vi "Mätning av ytresistivitet.vi"() -> ()   [LabVIEW 2024]
panel:
  out "Ytresistivitet, mWm":dbl
  out "Ytresistans, mW/*":dbl
  out "Mätvärden":dbl[][](array[numeric])
  out "% - max/min":dbl
  out "Max, Ytresistivitet":dbl
  out "Max, Ytresistans":dbl
  out "Min, Ytresistans":dbl
  out "Min, Ytresistivitet":dbl
  in  "Rensa sparade värden":bool
  in  "?":enum32{"Visa", "Göm"}(tab)
  out "Mätvärden2":dbl[][](array[numeric])
  out "% - skillnad":dbl
  out "Min":dbl format="%#_13g"
  out "Max":dbl
  out "Spänning.cal":dbl
  out "Ström.cal":dbl
  out "Redo för mätning3":bool
  out "Redo för mätning2":bool
  out "Redo för mätning":bool
  out "Mätning pågår":bool
  out "Kalibrering pågår":bool
  in  "Tab Control":T1(tab)
  in  "cal_onoff":bool caption="Boolean"
  in  "Sätt ström":bool
  in  "Nollställ ström":bool
  in  "Ange strömmen, mA":dbl
  in  "Kva/Lin":bool caption="Boolean"
  in  "Tjocklek, um":dbl
  in  "Material":string
  in  "Spänningsaggregat":refnum<visa-resource-name>="COM1"
  in  "Spänningsmultimeter":refnum<visa-resource-name>="USB0::0x0957::0x1B07::MY53100226::INSTR"
  in  "Strömmultimeter":refnum<visa-resource-name>="USB0::0x0957::0x1A07::MY53201212::INSTR"
  in  "Spara mätdata i textfil - linjärt":path
  in  "Spara mätdata i textfil - kvadratiskt":path
  in  "Spänning (V) +/- för kalibrering, default = 0,01V":dbl
  in  "Mapp för excelfiler":path=path "\\\\filur03.it.liu.se\\students/axefr422/Documents/Labview program/excel"
  in  "Samples/mätning, default = 10":i32
  in  "Max spänning (V), default = 1":dbl
  in  "Starta mätning":bool=TRUE
  in  "stop":bool
  # "Mätvärden"
  # "Medelvärden"
  # "Ytresistans, mW/*"
  # "Ytresistivitet, mWm"
  # "Specifik mätdata - Aktuell mätning"
  # "Spänning, V"
  # "Ström, A"
  # "Ytresistivitet, mWm"
  # "Ytresistans, mW/sq"
  # "Ytresistans"
  # "Kvadratiskt"
  # "Linjärt"
  # "Kalibrering av"
  # "Kalibrering på"
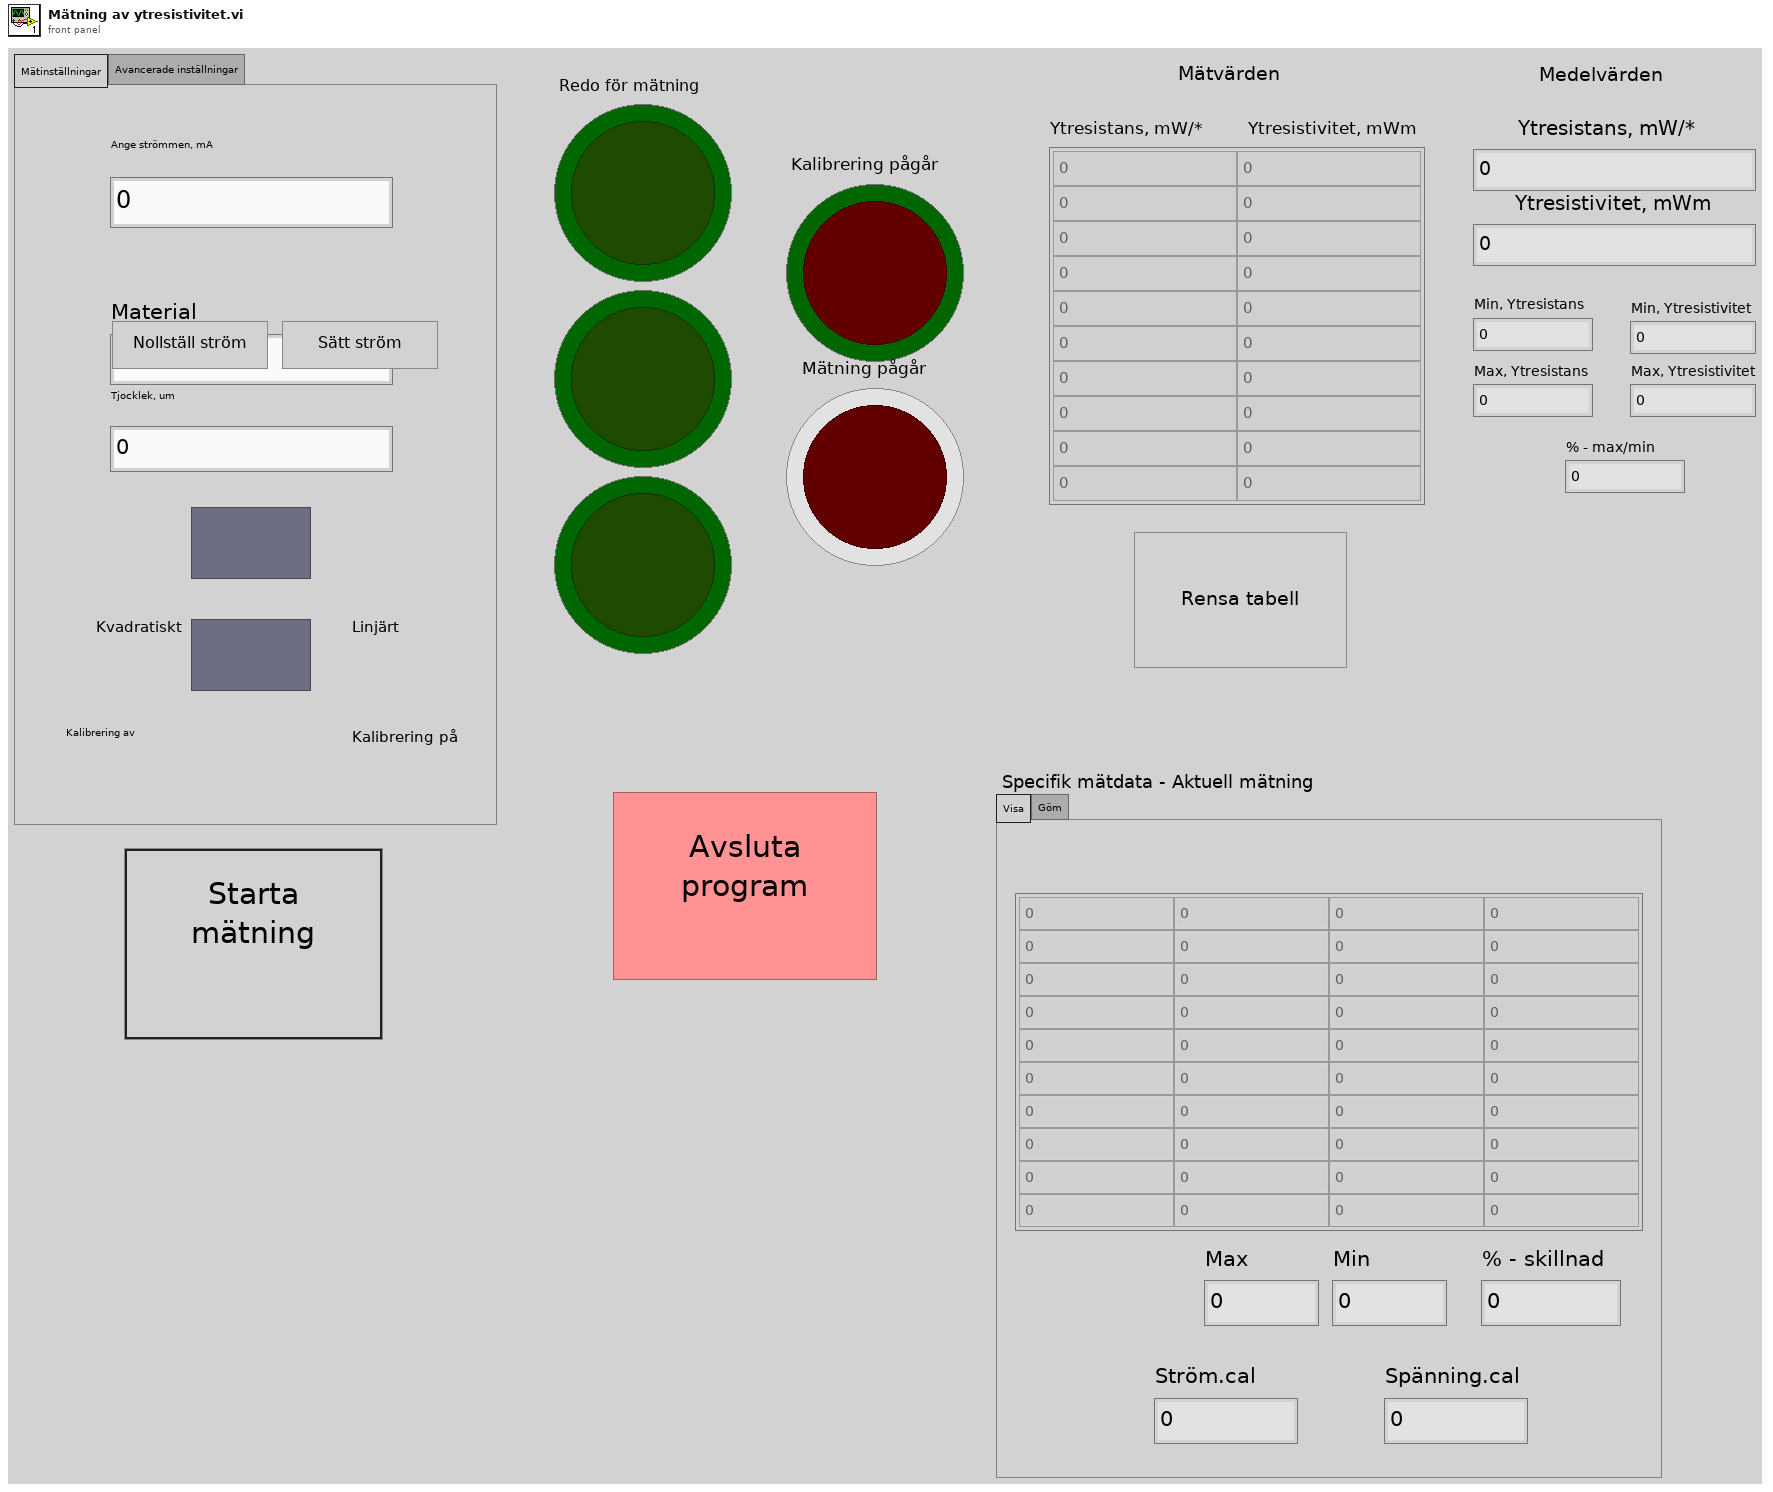
[diagram p1: front panel]
types:
  T1 = enum32{"Mätinställningar", "Avancerade inställningar"}
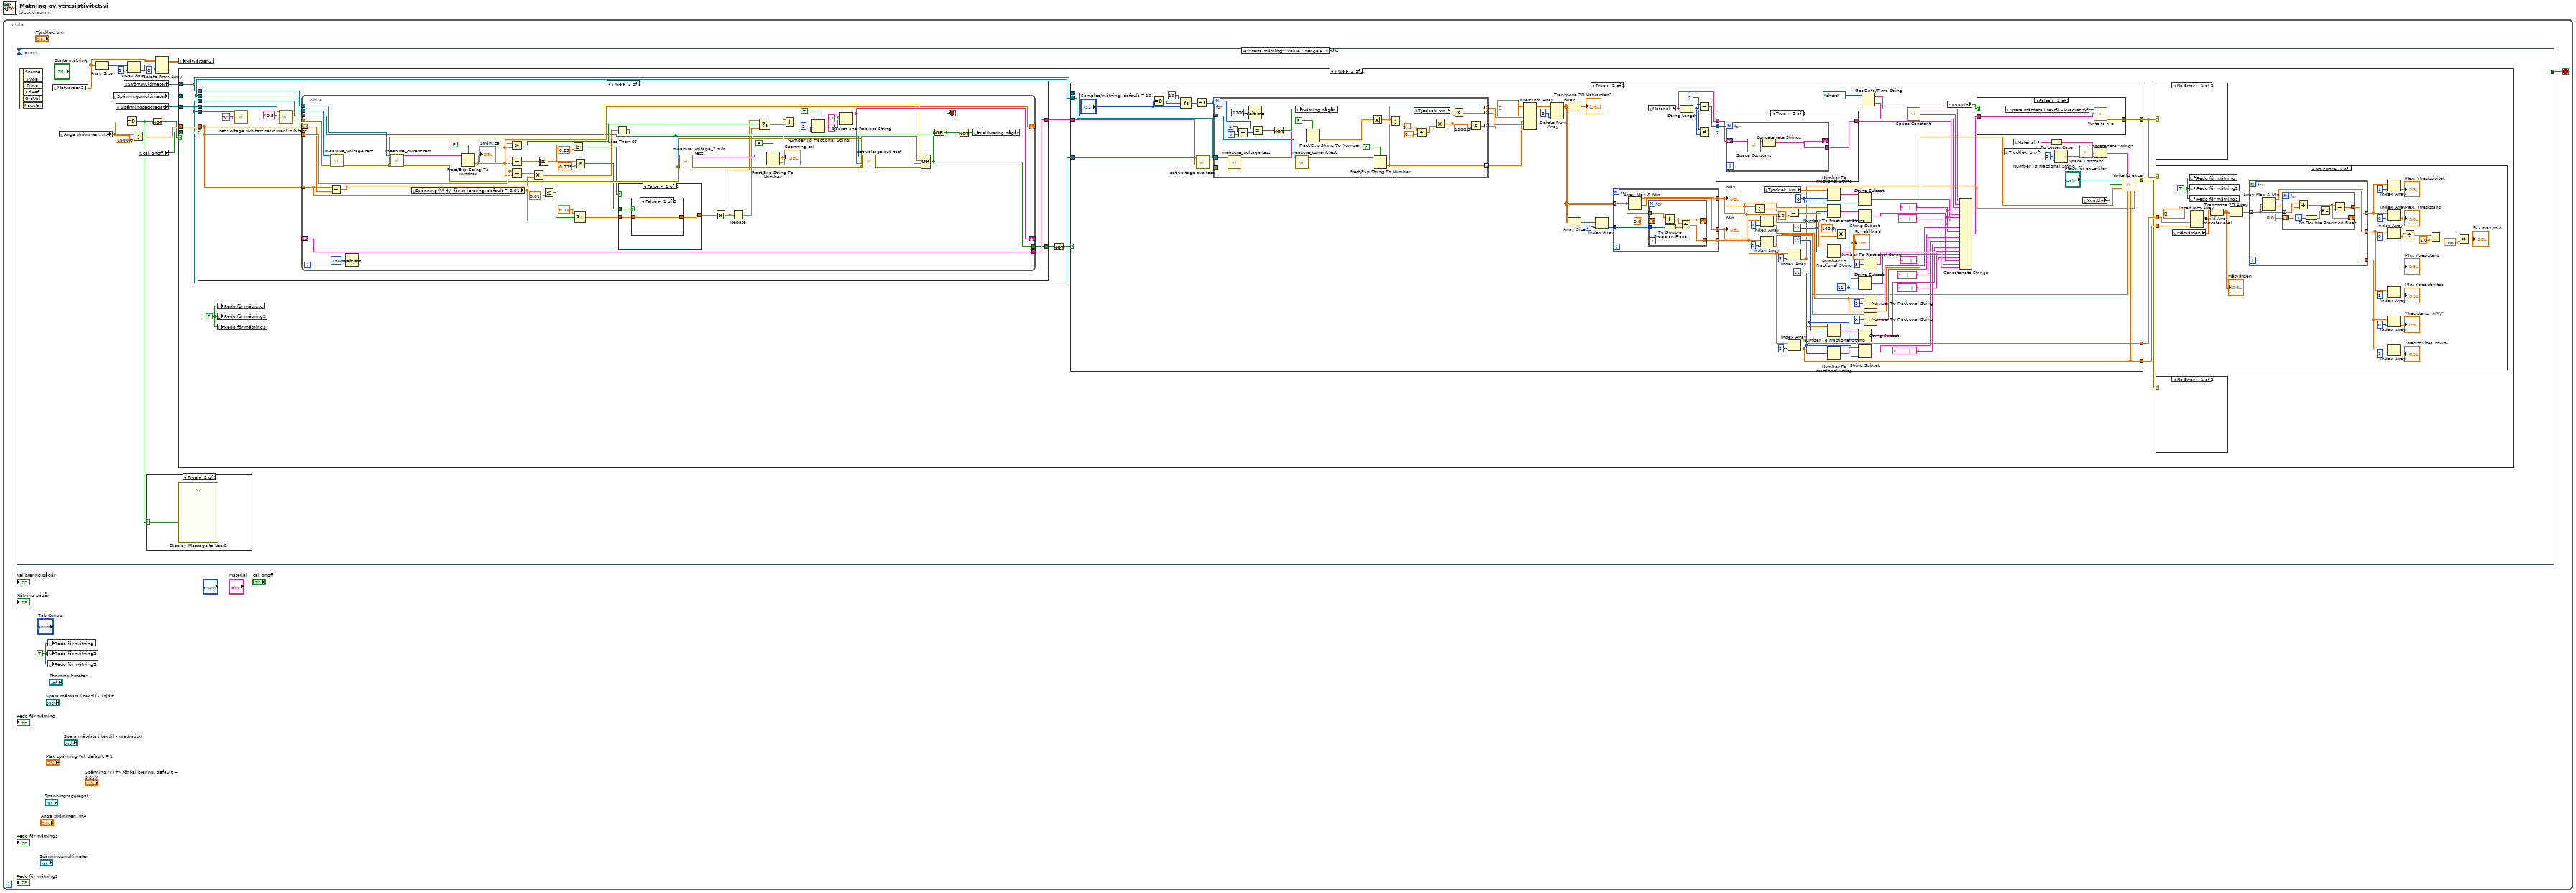
[diagram p0: block diagram]
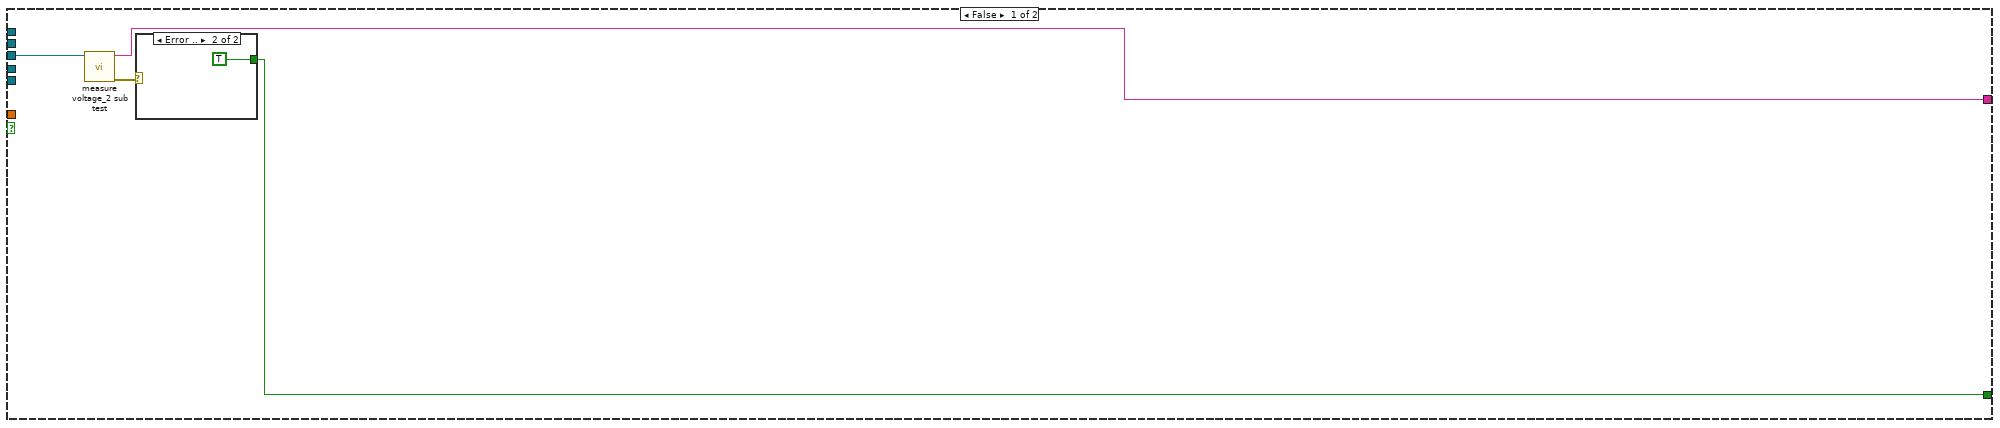
[diagram p4: hidden frame]
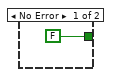
[diagram p5: hidden frame]
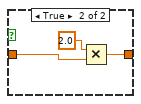
[diagram p6: hidden frame]
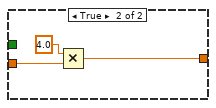
[diagram p7: hidden frame]
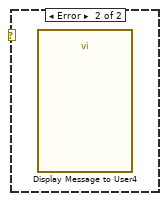
[diagram p8: hidden frame]
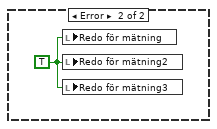
[diagram p9: hidden frame]
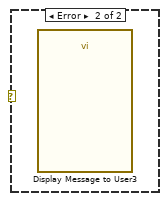
[diagram p10: hidden frame]
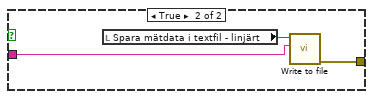
[diagram p12: hidden frame]
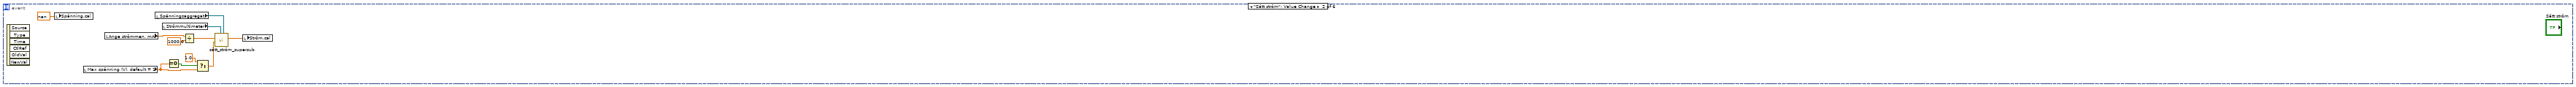
[diagram p14: hidden frame]
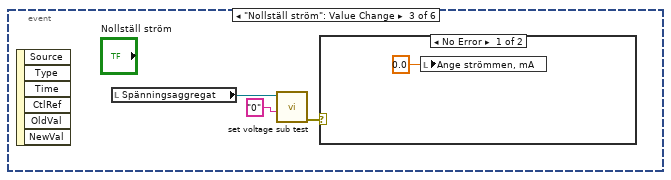
[diagram p15: hidden frame]
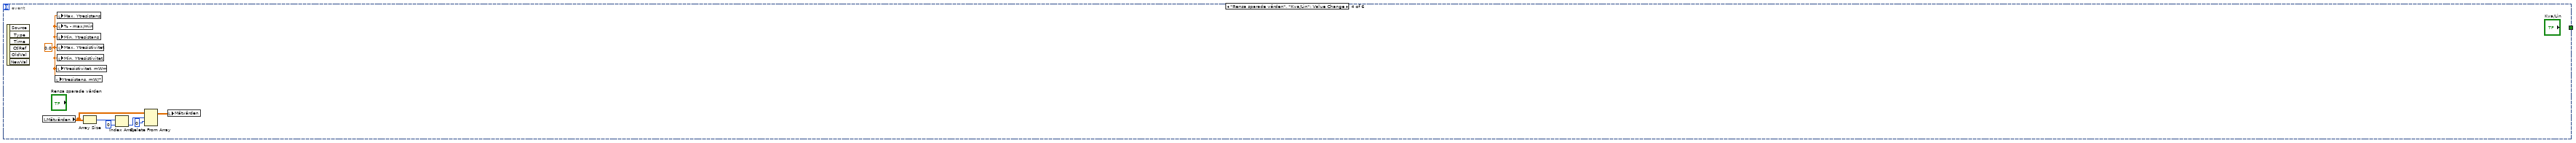
[diagram p17: hidden frame]
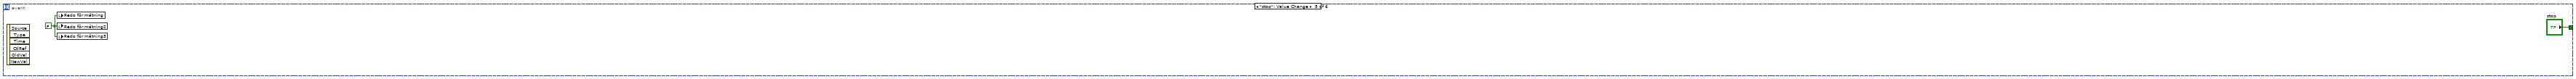
[diagram p18: hidden frame]
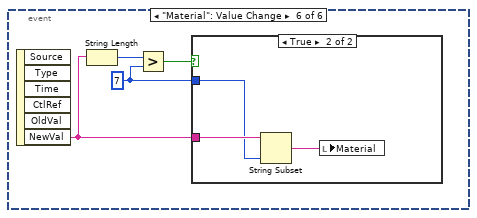
[diagram p19: hidden frame]
diagram:
  n1 = while {
    stop <- w2 stop-if-true
    w1 = TRUE ("Redo för mätning")
    n2 = event shown="[0] \"Starta mätning\": Value Change" {
      selector: _ -> [_ _ _ _ _ _]
      dyn-events: _ -> [_ _ _ _ _ _]
      timeout: _ -> [_ _ _ _ _ _]
      tunnel: [_ _ _ _ "stop" _] -> w2
      event "Starta mätning": Value Change {
        n3 = event-data() -> ()  [unwired: 1 in, 6 out]
        n4 = local read "Mätvärden2"() -> (w6:dbl[][])
        n5 = local read "Ange strömmen, mA"() -> (w12:dbl)
        n6 = Array Size(array=w6) -> (size(s)=w9:i32[])
        n7 = local read "Spänningsmultimeter"() -> (w14:refnum<visa-resource-name>)
        n8 = local read "Spänningsaggregat"() -> (w15:refnum<visa-resource-name>)
        n9 = local read "Strömmultimeter"() -> (w13:refnum<visa-resource-name>)
        n10 = Equal To 0?(x=w12) -> (x = 0?=w11:bool)
        n11 = Index Array(array=w9, index=0) -> (element=w7:i32)
        n12 = Divide(x=w12, y=1000.0) -> (x/y=w16:dbl)
        n13 = local read "cal_onoff"() -> (w3:bool)
        n14 = case shown="True" w11 {
          selector: w11 -> [_ w18]
          frame False {
          }
          frame True {
            n15 = call "Display Message to User2"("Enable"=w18) -> ()  [unwired: 9 in, 2 out]
          }
        }
        n16 = Not(x=w11) -> (.not. x?=w10:bool)
        n17 = Delete From Array(array=w6, length=w7, index (row)=0) -> (array with subset deleted=w5:dbl[][])  [unwired: 1 in, 1 out]
        n18 = local write "Mätvärden2"(w5) -> ()
        n19 = case shown="True" w10 {
          tunnel: w16 -> [_ w26]
          tunnel: w15 -> [_ w20]
          tunnel: w14 -> [_ w31]
          tunnel: w13 -> [_ w30]
          tunnel: w3 -> [_ w21]
          frame False {
          }
          frame True {
            w19 = FALSE ("Redo för mätning")
            n20 = case shown="True" w21 {
              tunnel: w31 -> [_ w49]
              tunnel: w30 -> [_ w48]
              tunnel: [w34 w47] -> w29
              tunnel: w20 -> [w35 w46]
              tunnel: [w32 w45] -> w28
              tunnel: w26 -> [_ w44]
              tunnel: w20 -> [_ w42]
              tunnel: w20 -> [_ w40]
              frame False {
                n21 = call "measure voltage_2 sub test.vi"("VISA Refnum in"=w35) -> ("error out"=w33:errorcluster, "Reponse"=w34:string)  [unwired: 9 in]
                n22 = case shown="Error .." w33 {
                  tunnel: [FALSE TRUE] -> w32
                  frame No Error {
                  }
                  frame Error {
                  }
                }
              }
              frame True {
                n23 = call "set voltage sub test.vi"("result string"="0", "VISA Refnum in"=w42) -> ("error out"=w43:errorcluster)  [unwired: 9 in]
                n24 = call "set current sub test.vi"("error in (no error)"=w43, "result string"="0.5", "VISA Refnum in"=w40) -> ("error out"=w39:errorcluster)  [unwired: 8 in]
                n25 = while {
                  tunnel: w44 -> [w98]
                  shift-right: [w67] -> _
                  shift-left: w44 -> [w96]
                  shift-right: [w97] -> _
                  shift-left: _ -> [w95]
                  tunnel: [w95] -> w47
                  tunnel: w46 -> [w51]
                  tunnel: w49 -> [w52]
                  tunnel: w48 -> [w76]
                  tunnel: [w70] -> w45
                  tunnel: w44 -> [w68]
                  tunnel: w39 -> [w50]
                  stop <- w71 stop-if-true
                  n26 = Subtract(x=w68, y=w96) -> (x-y=w85:dbl)
                  n27 = call "measure_voltage test.vi"("error in (no error)"=w50, "VISA Refnum in"=w52) -> ("error out"=w75:errorcluster)  [unwired: 8 in, 1 out]
                  n28 = Wait (ms)(milliseconds to wait=u32 750) -> ()  [unwired: 1 out]
                  n29 = call "measure_current test.vi"("error in (no error)"=w75, "VISA Refnum in"=w76) -> ("error out"=w74:errorcluster, "read buffer"=w78:string)  [unwired: 8 in]
                  n30 = local read "Spänning (V) +/- för kalibrering, default = 0,01V"() -> (w54:dbl)
                  n31 = Fract/Exp String To Number(use system decimal point (T)=FALSE, string=w78) -> (number=w67:dbl)  [unwired: 2 in, 1 out]
                  "Ström.cal" <- w67
                  n32 = Greater Or Equal?(x=w98, y=w67) -> (x >= y?=w92:bool)
                  n33 = Subtract(x=w68, y=w67) -> (x-y=w66:dbl)
                  n34 = Subtract(x=w68, y=w67) -> (x-y=w84:dbl)
                  n35 = Multiply(x=w84, y=w85) -> (x*y=w86:dbl)
                  n36 = Absolute Value(x=w66) -> (abs(x)=w58:dbl)
                  n37 = Less Or Equal?(x=w54, y=0.01) -> (x <= y?=w55:bool)
                  n38 = Greater Or Equal?(x=w58, y=0.25) -> (x >= y?=w64:bool)
                  n39 = Select(t=0.01, s=w55, f=w54) -> (s? t:f=w56:dbl)
                  n40 = Greater Or Equal?(x=w58, y=0.075) -> (x >= y?=w60:bool)
                  n41 = Less Than 0?(x=w86) -> (x < 0?=w72:bool)
                  n42 = case shown="False" w64 {
                    tunnel: w56 -> [w100 w108]
                    tunnel: [w99 w106] -> w63
                    tunnel: w60 -> [w101 _]
                    frame False {
                      n43 = case shown="False" w101 {
                        tunnel: w100 -> [w102 w104]
                        tunnel: [w102 w103] -> w99
                        frame False {
                        }
                        frame True {
                          n44 = Multiply(x=2.0, y=w104) -> (x*y=w103:dbl)
                        }
                      }
                    }
                    frame True {
                      n45 = Multiply(x=4.0, y=w108) -> (x*y=w106:dbl)
                    }
                  }
                  n46 = call "measure voltage_2 sub test.vi"("error in (no error)"=w74, "VISA Refnum in"=w51) -> ("error out"=w73:errorcluster, "Reponse"=w79:string)  [unwired: 8 in]
                  n47 = Absolute Value(x=w63) -> (abs(x)=w61:dbl)
                  n48 = Negate(x=w61) -> (-x=w62:dbl)
                  n49 = Select(t=w61, s=w92, f=w62) -> (s? t:f=w91:dbl)
                  n50 = Fract/Exp String To Number(use system decimal point (T)=FALSE, string=w79) -> (number=w81:dbl)  [unwired: 2 in, 1 out]
                  "Spänning.cal" <- w81
                  n51 = Add(x=w81, y=w91) -> (x+y=w83:dbl)
                  n52 = Number To Fractional String(use system decimal point (T)=TRUE, number=w83, precision (6)=i16 2) -> (F-format string=w82:string)  [unwired: 1 in]
                  n53 = Search and Replace String(input string=w82, search string=",", replace string="." ("replace string (\"\")")) -> (result string=w97:string)  [unwired: 5 in, 3 out]
                  n54 = call "set voltage sub test.vi"("error in (no error)"=w73, "result string"=w97, "VISA Refnum in"=w51) -> ("error out"=w69:errorcluster)  [unwired: 8 in]
                  n55 = Compound Arithmetic op=OR(w75, w74, w73, w69) -> (w70:bool)
                  n56 = Or(x=w70, y=w72) -> (x .or. y?=w71:bool)
                  n57 = Not(x=w71) -> (.not. x?=w77:bool)
                  n58 = local write "Kalibrering pågår"(w77) -> ()
                }
              }
            }
            n59 = local write "Redo för mätning"(w19) -> ()
            n60 = local write "Redo för mätning2"(w19) -> ()
            n61 = local write "Redo för mätning3"(w19) -> ()
            n62 = Not(x=w28) -> (.not. x?=w27:bool)
            n63 = case shown="True" w27 {
              tunnel: w31 -> [_ w179]
              tunnel: w30 -> [_ w178]
              tunnel: w29 -> [_ w177]
              tunnel: w20 -> [_ w176]
              tunnel: [_ w174] -> w25
              tunnel: [_ w162] -> w23
              tunnel: [_ w161] -> w24
              tunnel: [_ w158] -> w22
              frame False {
              }
              frame True {
                w175 = i16 8 ("width (-)")
                w203 = i16 11 ("width (-)")
                w200 = i16 11 ("width (-)")
                w201 = 7 ("x")
                w199 = 11 ("length (rest)")
                w196 = i16 11 ("width (-)")
                w190 = "    |    "
                n64 = Equal To 0?(x="Samples/mätning, default = 10") -> (x = 0?=w156:bool)
                n65 = Select(t=10, s=w156, f="Samples/mätning, default = 10") -> (s? t:f=w153:i32)
                n66 = Increment(x=w153) -> (x+1=w157:i32)
                n67 = call "set voltage sub test.vi"("result string"=w177, "VISA Refnum in"=w176) -> ("error out"=w206:errorcluster)  [unwired: 9 in]
                n68 = for {
                  N: w157 -> [w282]
                  tunnel: [w269] -> w204 mode=indexing
                  tunnel: [w287] -> w205 mode=indexing
                  tunnel: w206 -> [w284]
                  tunnel: w179 -> [w276]
                  tunnel: w178 -> [w275]
                  tunnel: [w271] -> w221 mode=indexing
                  tunnel: [w264] -> w232 mode=indexing
                  i -> [w281]
                  n69 = call "measure_voltage test.vi"("error in (no error)"=w284, "VISA Refnum in"=w276) -> ("error out"=w283:errorcluster, "read buffer"=w285:string)  [unwired: 8 in]
                  n70 = Add(x=1, y=w281) -> (x+y=w277:i32)
                  n71 = Wait (ms)(milliseconds to wait=u32 1000) -> ()  [unwired: 1 out]
                  n72 = Equal?(x=w282, y=w277) -> (x = y?=w279:bool)
                  n73 = Not(x=w279) -> (.not. x?=w278:bool)
                  n74 = local write "Mätning pågår"(w278) -> ()
                  n75 = call "measure_current test.vi"("error in (no error)"=w283, "VISA Refnum in"=w275) -> ("read buffer"=w286:string)  [unwired: 8 in, 1 out]
                  n76 = Fract/Exp String To Number(use system decimal point (T)=FALSE, string=w285) -> (number=w270:dbl)  [unwired: 2 in, 1 out]
                  n77 = Absolute Value(x=w270) -> (abs(x)=w269:dbl)
                  n78 = Fract/Exp String To Number(use system decimal point (T)=FALSE, string=w286) -> (number=w287:dbl)  [unwired: 2 in, 1 out]
                  n79 = Divide(x=w269, y=w287) -> (x/y=w268:dbl)
                  n80 = local read "Tjocklek, um"() -> (w267:dbl)
                  n81 = Divide(x=3.141592653589793, y=0.6931471805599453) -> (x/y=w274:dbl)
                  n82 = Multiply(x=w268, y=w274) -> (x*y=w265:dbl)
                  n83 = Multiply(x=w267, y=w265) -> (x*y=w271:dbl)
                  n84 = Multiply(x=w265, y=1000.0) -> (x*y=w264:dbl)
                }
                n85 = Insert Into Array(array=dbl[][] [], new element #1=w204, new element #2=w205, new element #3=w221, new element #4=w232) -> (w207:dbl[][])  [unwired: 2 in]
                n86 = Delete From Array(array=w207, index (col)=0) -> (array with subset deleted=w215:dbl[][])  [unwired: 2 in, 1 out]
                n87 = Transpose 2D Array(2D array=w215) -> (transposed array=→"Mätvärden2":dbl[][])
                n88 = Array Size(array=w215) -> (size(s)=w208:i32[])
                n89 = Index Array(array=w208, index=1) -> (element=w209:i32)
                n90 = for {
                  tunnel: [w257] -> w234 mode=indexing
                  tunnel: w215 -> [w254] mode=indexing
                  tunnel: w209 -> [w255]
                  tunnel: [w253] -> w152
                  tunnel: [w252] -> w151
                  n91 = Array Max & Min(array=w254) -> (max value=w253:dbl, min value=w252:dbl)  [unwired: 2 out]
                  n92 = for {
                    tunnel: [w258] -> w257
                    shift-right: [w263] -> _
                    shift-left: 0.0 -> [w262]
                    tunnel: w254 -> [w260] mode=indexing
                    tunnel: w255 -> [w259]
                    n93 = Add(x=w260, y=w262) -> (x+y=w263:dbl)
                    n94 = To Double Precision Float(number=w259) -> (double precision float=w261:dbl)
                    n95 = Divide(x=w263, y=w261) -> (x/y=w258:dbl)
                  }
                }
                "Max" <- w152
                "Min" <- w151
                n96 = local read "Material"() -> (w227:string)
                n97 = String Length(string=w227) -> (length=w231:i32)
                n98 = Subtract(x=w201, y=w231) -> (x-y=w230:i32)
                n99 = Not Equal?(x=w201, y=w231) -> (x != y?=w229:bool)
                n100 = case shown="True" w229 {
                  tunnel: w230 -> [_ w248]
                  tunnel: w227 -> [w245 w247]
                  tunnel: [w245 w246] -> w228
                  frame False {
                  }
                  frame True {
                    n101 = for {
                      N: w248 -> [_]
                      shift-right: [w249] -> _
                      shift-left: w247 -> [w250]
                      tunnel: [w249] -> w246
                      n102 = call <vilib>:"Space Constant.vi"() -> ("String"=w251:string)
                      n103 = Concatenate Strings(w250, w251) -> (w249:string)
                    }
                  }
                }
                n104 = Divide(x=w152, y=w151) -> (x/y=w210:dbl)
                n105 = Index Array(array=w234, index=0) -> (element=w171:dbl)
                n106 = Index Array(array=w234, index=1) -> (element=w170:dbl)
                n107 = local read "Tjocklek, um"() -> (w222:dbl)
                n108 = Subtract(x=w210, y=1.0) -> (x-y=w214:dbl)
                n109 = Index Array(array=w234, index=3) -> (element=w162:dbl)
                n110 = Index Array(array=w234, index=2) -> (element=w161:dbl)
                n111 = Number To Fractional String(number=w222, precision (6)=w175) -> (F-format string=w223:string)  [unwired: 2 in]
                n112 = Number To Fractional String(number=w152, width (-)=w196) -> (F-format string=w218:string)  [unwired: 2 in]
                n113 = Number To Fractional String(number=w151, width (-)=w196) -> (F-format string=w217:string)  [unwired: 2 in]
                n114 = Number To Fractional String(number=w162, width (-)=w203) -> (F-format string=w233:string)  [unwired: 2 in]
                n115 = Number To Fractional String(number=w161, width (-)=w200) -> (F-format string=w219:string)  [unwired: 2 in]
                n116 = Multiply(x=100.0, y=w214) -> (x*y=w150:dbl)
                "% - skillnad" <- w150
                n117 = String Subset(string=w223, length (rest)=w175) -> (substring=w173:string)  [unwired: 1 in]
                n118 = String Subset(string=w218, length (rest)=w199) -> (substring=w237:string)  [unwired: 1 in]
                n119 = String Subset(string=w217, length (rest)=w199) -> (substring=w236:string)  [unwired: 1 in]
                n120 = String Subset(string=w233, length (rest)=w203) -> (substring=w235:string)  [unwired: 1 in]
                n121 = String Subset(string=w219, length (rest)=w200) -> (substring=w220:string)  [unwired: 1 in]
                n122 = Get Date/Time String(date format (0)=enum16{"short", "long", "abbreviated"}."short") -> (date string=w224:string, time string=w226:string)  [unwired: 2 in]
                n123 = Number To Fractional String(number=w150, width (-)=i16 8) -> (F-format string=w238:string)  [unwired: 2 in]
                n124 = Number To Fractional String(number=w171, width (-)=i16 9) -> (F-format string=w212:string)  [unwired: 2 in]
                n125 = Number To Fractional String(number=w170, width (-)=i16 8) -> (F-format string=w213:string)  [unwired: 2 in]
                n126 = call <vilib>:"Space Constant.vi"() -> ("String"=w225:string)
                n127 = local read "Kva/Lin"() -> (w160:bool)
                n128 = Concatenate Strings(w224, w225, w226, w190, w228, w190, w173, w190, w212, w190, w213, "    |      ", w220, "         |     ", w235, "       |   " ("string"), w236, "     |   " ("string"), w237, "     |    " ("string"), w238) -> (w211:string)
                n129 = case shown="False" w160 {
                  tunnel: w211 -> [w241 w243]
                  tunnel: [w239 w242] -> w174
                  frame False {
                    n130 = local read "Spara mätdata i textfil - kvadratiskt"() -> (w240:path)
                    n131 = call "Write to file.vi"("input string"=w241, "file path"=w240) -> ("error out"=w239:errorcluster)  [unwired: 9 in]
                  }
                  frame True {
                    n132 = local read "Spara mätdata i textfil - linjärt"() -> (w244:path)
                    n133 = call "Write to file.vi"("input string"=w243, "file path"=w244) -> ("error out"=w242:errorcluster)  [unwired: 9 in]
                  }
                }
                n134 = local read "Tjocklek, um"() -> (w165:dbl)
                n135 = local read "Material"() -> (w168:string)
                n136 = To Lower Case(string=w168) -> (all lower case string=w169:string)
                n137 = Number To Fractional String(number=w165, precision (6)=i16 2) -> (F-format string=w163:string)  [unwired: 2 in]
                n138 = call <vilib>:"Space Constant.vi"() -> ("String"=w166:string)
                n139 = local read "Kva/Lin"() -> (w159:bool)
                n140 = Concatenate Strings(w169, w166, w163) -> (w172:string)
                n141 = call "Write to excel.vi"("Mapp"="Mapp för excelfiler", "Filnamn"=w172, "Boolean"=w159, "Spänning"=w171, "Ström"=w170, "Ytresistivitet"=w161, "Ytresistans"=w162) -> ("error out"=w158:errorcluster)  [unwired: 2 in]
              }
            }
            n142 = case shown="No Error" w25 {
              frame No Error {
              }
              frame Error {
                n143 = call "Display Message to User3"() -> ()  [unwired: 10 in, 2 out]
              }
            }
            n144 = case shown="No Error" w25 {
              tunnel: w24 -> [w130 _]
              tunnel: w23 -> [w131 _]
              frame No Error {
                w109 = TRUE ("Redo för mätning")
                n145 = local read "Mätvärden"() -> (w128:dbl[][])
                n146 = local write "Redo för mätning"(w109) -> ()
                n147 = local write "Redo för mätning2"(w109) -> ()
                n148 = local write "Redo för mätning3"(w109) -> ()
                n149 = Insert Into Array(array=dbl[] [], new element #1=w131, new element #2=w130) -> (w127:dbl[])  [unwired: 1 in]
                n150 = Build Array (concatenate)(w128, w127) -> (w126:dbl[][])
                "Mätvärden" <- w126
                n151 = Transpose 2D Array(2D array=w126) -> (transposed array=w125:dbl[][])
                n152 = for {
                  tunnel: [w140] -> w134 mode=indexing
                  tunnel: w125 -> [w139] mode=indexing
                  tunnel: [w138] -> w123 mode=indexing
                  tunnel: [w137] -> w124 mode=indexing
                  n153 = Array Max & Min(array=w139) -> (max value=w138:dbl, min value=w137:dbl)  [unwired: 2 out]
                  n154 = for {
                    shift-right: [w145] -> _
                    shift-left: 0.0 -> [w148]
                    tunnel: [w146] -> w140
                    tunnel: w139 -> [w144] mode=indexing
                    i -> [w147]
                    n155 = Add(x=w144, y=w148) -> (x+y=w145:dbl)
                    n156 = To Double Precision Float(number=w147) -> (double precision float=w143:dbl)
                    n157 = Increment(x=w143) -> (x+1=w142:dbl)
                    n158 = Divide(x=w145, y=w142) -> (x/y=w146:dbl)
                  }
                }
                n159 = Index Array(array=w123, index=1) -> (element=→"Max, Ytresistivitet":dbl)
                n160 = Index Array(array=w123, index=0) -> (element=w118:dbl)
                "Max, Ytresistans" <- w118
                n161 = Index Array(array=w124, index=0) -> (element=w117:dbl)
                "Min, Ytresistans" <- w117
                n162 = Index Array(array=w124, index=1) -> (element=→"Min, Ytresistivitet":dbl)
                n163 = Index Array(array=w134, index=0) -> (element=→"Ytresistans, mW/*":dbl)
                n164 = Index Array(array=w134, index=1) -> (element=→"Ytresistivitet, mWm":dbl)
                n165 = Divide(x=w118, y=w117) -> (x/y=w116:dbl)
                n166 = Subtract(x=w116, y=1.0) -> (x-y=w114:dbl)
                n167 = Multiply(x=w114, y=100.0) -> (x*y=→"% - max/min":dbl)
              }
              frame Error {
                w149 = TRUE ("Redo för mätning3")
                n168 = local write "Redo för mätning"(w149) -> ()
                n169 = local write "Redo för mätning2"(w149) -> ()
                n170 = local write "Redo för mätning3"(w149) -> ()
              }
            }
            n171 = case shown="No Error" w22 {
              frame No Error {
              }
              frame Error {
                n172 = call "Display Message to User4"() -> ()  [unwired: 10 in, 2 out]
              }
            }
          }
        }
      }
      event "Sätt ström": Value Change {
        n173 = event-data() -> ()  [unwired: 1 in, 6 out]
        n174 = local write "Spänning.cal"(nan ("Spänning.cal")) -> ()
        n175 = local read "Max spänning (V), default = 1"() -> (w295:dbl)
        n176 = local read "Ange strömmen, mA"() -> (w300:dbl)
        n177 = local read "Spänningsaggregat"() -> (w293:refnum<visa-resource-name>)
        n178 = local read "Strömmultimeter"() -> (w301:refnum<visa-resource-name>)
        n179 = Equal To 0?(x=w295) -> (x = 0?=w297:bool)
        n180 = Divide(x=w300, y=1000.0) -> (x/y=w298:dbl)
        n181 = Select(t=1.0, s=w297, f=w295) -> (s? t:f=w294:dbl)
        n182 = call "sätt_ström_supersub.vi"("Spänningsaggregat"=w293, "Strömmultimeter"=w301, "voltage_max"=w294, "current_in"=w298) -> ("current_act"=w292:dbl)  [unwired: 6 in, 1 out]
        n183 = local write "Ström.cal"(w292) -> ()
      }
      event "Nollställ ström": Value Change {
        n184 = event-data() -> ()  [unwired: 1 in, 6 out]
        n185 = local read "Spänningsaggregat"() -> (w304:refnum<visa-resource-name>)
        n186 = call "set voltage sub test.vi"("result string"="0", "VISA Refnum in"=w304) -> ("error out"=w302:errorcluster)  [unwired: 9 in]
        n187 = case shown="No Error" w302 {
          frame No Error {
            n188 = local write "Ange strömmen, mA"(0.0 ("Ström")) -> ()
          }
          frame Error {
          }
        }
      }
      event "Rensa sparade värden", "Kva/Lin": Value Change {
        w306 = 0.0 ("Ytresistans")
        n189 = event-data() -> ()  [unwired: 1 in, 6 out]
        n190 = local read "Mätvärden"() -> (w312:dbl[][])
        n191 = local write "Ytresistans, mW/*"(w306) -> ()
        n192 = local write "Ytresistivitet, mWm"(w306) -> ()
        n193 = local write "Max, Ytresistans"(w306) -> ()
        n194 = local write "% - max/min"(w306) -> ()
        n195 = local write "Min, Ytresistans"(w306) -> ()
        n196 = local write "Max, Ytresistivitet"(w306) -> ()
        n197 = local write "Min, Ytresistivitet"(w306) -> ()
        n198 = Array Size(array=w312) -> (size(s)=w310:i32[])
        n199 = Index Array(array=w310, index=0) -> (element=w308:i32)
        n200 = Delete From Array(array=w312, length=w308, index (row)=0) -> (array with subset deleted=w311:dbl[][])  [unwired: 1 in, 1 out]
        n201 = local write "Mätvärden"(w311) -> ()
      }
      event "stop": Value Change {
        w313 = FALSE ("Redo för mätning")
        n202 = event-data() -> ()  [unwired: 1 in, 6 out]
        n203 = local write "Redo för mätning"(w313) -> ()
        n204 = local write "Redo för mätning2"(w313) -> ()
        n205 = local write "Redo för mätning3"(w313) -> ()
      }
      event "Material": Value Change {
        w315 = 7 ("y")
        n206 = event-data() -> ("NewVal"=w318:string)  [unwired: 1 in, 5 out]
        n207 = String Length(string=w318) -> (length=w317:i32)
        n208 = Greater?(x=w317, y=w315) -> (0:w316:bool)
        n209 = case shown="True" w316 {
          tunnel: w318 -> [_ w320]
          tunnel: w315 -> [_ w319]
          frame False {
          }
          frame True {
            n210 = String Subset(string=w320, length (rest)=w319) -> (substring=w321:string)  [unwired: 1 in]
            n211 = local write "Material"(w321) -> ()
          }
        }
      }
    }
    n212 = local write "Redo för mätning"(w1) -> ()
    n213 = local write "Redo för mätning2"(w1) -> ()
    n214 = local write "Redo för mätning3"(w1) -> ()
  }
